vi "Word Report - Multiple Pages.vi"   [LabVIEW 2023]
doc: "This example shows how to generate a series of Word document reports and an index table that contains links to the individual reports.\n\nTo execute this example, select a directory in which you want to save the reports and click the Run button."
uses:
  <vilib>/Utility/NIReport.llb/Report Type.ctl
  <vilib>/Utility/NIReport.llb/Append Report Text (str wrap).vi
  <vilib>/Utility/NIReport.llb/NI_report.lvclass
  <vilib>/Utility/NIReport.llb/Word/NI_Word.lvclass
  <vilib>/Utility/NIReport.llb/NI_ReportGenerationCore.lvlib
panel:
  # "Overview: This example shows how to generate a series of reports and an index table that contains links to the individual reports.\nRequirements: Report Generation Toolkit, Microsoft Word\nInstructions:\n1. Close Microsoft Word before starting the VI.\n2. Run the VI.\n\nNote: The Word documents generated by this example are saved in the <LabVIEW Data> Folder."
types:
  T1 = typedef "NI_ReportGenerationCore.lvlib/Report Type.ctl" = enum16{"HTML", "Word", "Excel"}
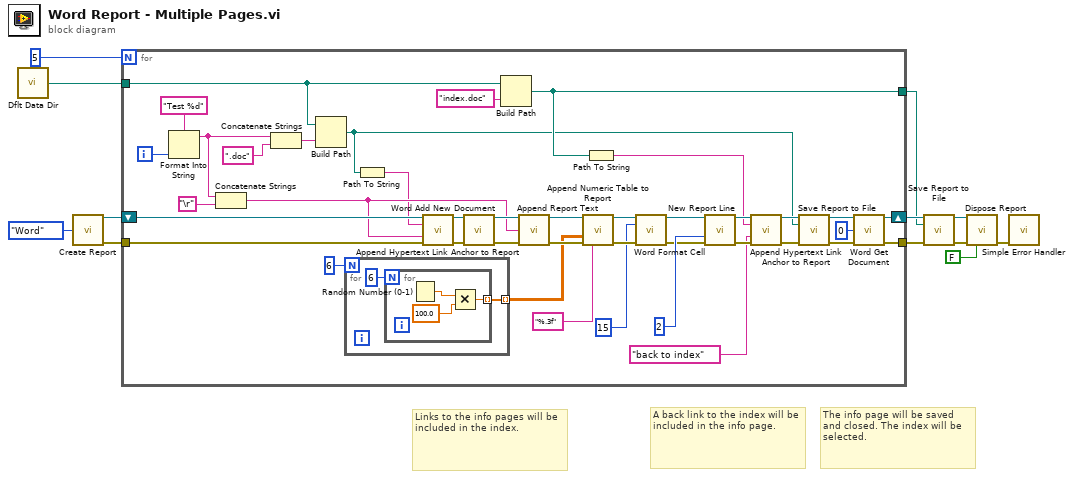
[diagram p0: block diagram]
diagram:
  # "The info page will be saved and closed. The index will be selected."
  # "A back link to the index will be included in the info page."
  # "Links to the info pages will be included in the index."
  n1 = call <vilib>:"Dflt Data Dir.vi"() -> ("App:Default Data Directory"=w2:path)
  n2 = call <vilib>:"Create Report.vi"("report type"=Report_Type."Word" ("Report Type")) -> ("report out"=w10:refnum<class "NI_report.lvclass">, "error out"=w12:errorcluster)  [unwired: 13 in]
  n3 = for {
    N: 5 -> [_]
    tunnel: w12 -> [w38]
    tunnel: [w50] -> w7
    shift-right: [w49] -> w6
    shift-left: w10 -> [w37]
    tunnel: [w35] -> w5
    tunnel: w2 -> [w15]
    i -> [w32]
    n4 = Format Into String(format string="Test %d" ("Input String"), w32) -> (resulting string=w18:string)  [unwired: 2 in, 1 out]
    n5 = Concatenate Strings(w18, "\r") -> (w19:string)
    n6 = Concatenate Strings(w18, ".doc" ("Substring")) -> (w16:string)
    n7 = Build Path(base path=w15, name or relative path=w16) -> (appended path=w13:path)
    n8 = for {
      N: 6 -> [_]
      tunnel: [w53] -> w22 mode=indexing
      n9 = for {
        N: 6 ("dimension size") -> [_]
        tunnel: [w55] -> w53 mode=indexing
        n10 = Random Number (0-1)() -> (number: 0 to 1=w57:dbl)
        n11 = Multiply(x=w57, y=100.0) -> (x*y=w55:dbl)
      }
    }
    n12 = Path To String(path=w13) -> (string=w14:string)
    n13 = call-dynamic "Append Hypertext Link Anchor to Report.vi"("report in"=w37, "URL of link - href"=w14, "link text"=w19, "error in (no error)"=w38) -> ("report out"=w51:refnum<class "NI_report.lvclass">, "error out"=w52:errorcluster)  [unwired: 8 in, 2 out]
    n14 = call <vilib>:"Word Add New Document.vi"("report in"=w51, "error in (no error)"=w52) -> ("report out"=w47:refnum<class "NI_report.lvclass">, "error out"=w48:errorcluster)  [unwired: 12 in]
    n15 = Build Path(base path=w15, name or relative path="index.doc") -> (appended path=w35:path)
    n16 = call-poly <vilib>:"Append Report Text.vi"("report in"=w47, "text"=w19, "error in (no error)"=w48) -> ("report out"=w45:refnum<class "NI_report.lvclass">, "error out"=w46:errorcluster)  [unwired: 9 in, 2 out]
    n17 = call-dynamic "Append Numeric Table to Report.vi"("report in"=w45, "numerical data"=w22, "error in (no error)"=w46, "format string (%.3f)"="%.3f" ("format string")) -> ("report out"=w41:refnum<class "NI_report.lvclass">, "error out"=w43:errorcluster)  [unwired: 8 in, 2 out]
    n18 = Path To String(path=w35) -> (string=w24:string)
    n19 = call <vilib>:"Word Format Cell.vi"("report in"=w41, "autoformat (-1: none)"=i16 15 ("autoformat"), "error in (no error)"=w43) -> ("report out"=w40:refnum<class "NI_report.lvclass">, "error out"=w42:errorcluster)  [unwired: 11 in]
    n20 = call-dynamic "New Report Line.vi"("report in"=w40, "number of lines (1)"=2 ("number of lines"), "error in (no error)"=w42) -> ("report out"=w28:refnum<class "NI_report.lvclass">, "error out"=w29:errorcluster)  [unwired: 11 in]
    n21 = call-dynamic "Append Hypertext Link Anchor to Report.vi"("report in"=w28, "URL of link - href"=w24, "link text"="back to index", "error in (no error)"=w29) -> ("report out"=w27:refnum<class "NI_report.lvclass">, "error out"=w26:errorcluster)  [unwired: 8 in, 2 out]
    n22 = call-dynamic "Save Report to File.vi"("report in"=w27, "report file path"=w13, "error in (no error)"=w26) -> ("report out"=w31:refnum<class "NI_report.lvclass">, "error out"=w30:errorcluster)  [unwired: 11 in]
    n23 = call <vilib>:"Word Get Document.vi"("report in"=w31, "document index (0)"=0, "error in (no error)"=w30) -> ("report out"=w49:refnum<class "NI_report.lvclass">, "error out"=w50:errorcluster)  [unwired: 11 in]
  }
  n24 = call-dynamic "Save Report to File.vi"("report in"=w6, "report file path"=w5, "error in (no error)"=w7) -> ("report out"=w8:refnum<class "NI_report.lvclass">, "error out"=w9:errorcluster)  [unwired: 11 in]
  n25 = call-dynamic "Dispose Report.vi"("report in"=w8, "error in (no error)"=w9, "close report? (T)"=FALSE ("Close Report? (T)")) -> ("error out"=w4:errorcluster)  [unwired: 12 in]
  n26 = call <vilib>:"Simple Error Handler.vi"("error in (no error)"=w4) -> ()  [unwired: 4 in, 5 out]
